vi "dfd_Format Number.vi"(7 "format string":string, 11 "Coefficient":dbl) -> (3 "String Coefficient":string)   [LabVIEW 2017, in "NI_DigFilter_Process.lvlib"]
uses:
  <vilib>/addons/Digital Filter Design/NI_DigFilter_Process.lvlib
panel:
  out "output string":string
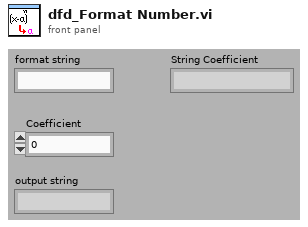
[diagram p1: front panel]
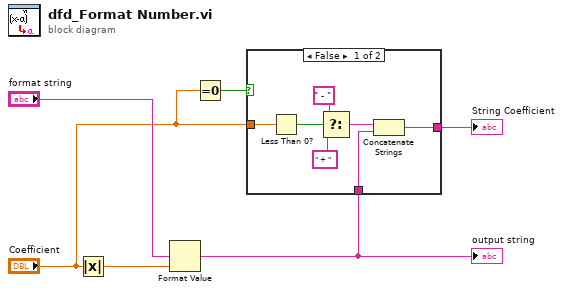
[diagram p0: block diagram]
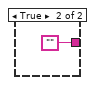
[diagram p2: hidden frame]
diagram:
  n1 = Absolute Value(x="Coefficient") -> (abs(x)=w5:dbl)
  n2 = Format Value(format string="format string", value (0)=w5) -> (output string=w1:string)  [unwired: 1 out]
  "output string" <- w1
  n3 = Equal To 0?(x="Coefficient") -> (x = 0?=w2:bool)
  n4 = case shown="False" w2 {
    tunnel: [w11 ""] -> w6
    tunnel: w1 -> [w8 _]
    tunnel: "Coefficient" -> [w7 _]
    frame False {
      n5 = Less Than 0?(x=w7) -> (x < 0?=w12:bool)
      n6 = Select(t=" - " ("string"), s=w12, f=" + ") -> (s? t:f=w10:string)
      n7 = Concatenate Strings(w10, w8) -> (w11:string)
    }
    frame True {
    }
  }
  "String Coefficient" <- w6
